vi "API_Get Current Position.vi"(10 "STATUS cluster":T1) -> (1 "Connected":bool, 3 "Probe Position":dbl)   [LabVIEW 2015, in "Tool Module.lvlib"]
doc: "Take the provided Tool Module Status cluster and extract the current axial position. Also output the current connection status. This is used to enable or disable and grayout the position display.\n\nThis vi can be used with the Tool STATUS cluster sent as the payload of the Tool Module Broadcast Event.Send Status User Event.\n\n<b>Note:</b> This VI was modified by the <b>Validate DQMH Module</b> tool to turn off automatic error handling."
uses:
  Tool Module.lvlib
  Support/_STATUS Typedef--cluster.ctl
  Tool Config/Tool Cfg.lvlib
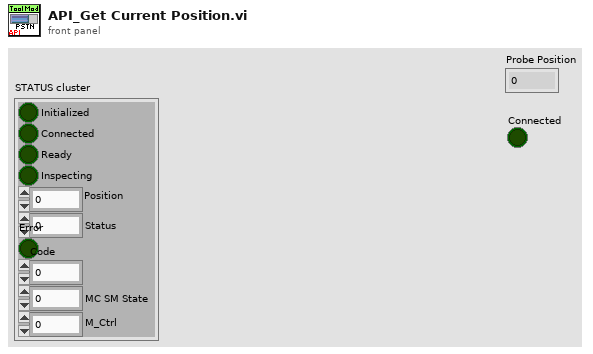
[diagram p1: front panel]
types:
  T1 = typedef "Tool Module.lvlib/_STATUS Typedef--cluster.ctl" = cluster{"Initialized":bool, "Connected":bool, "Ready":bool, "Inspecting":bool, "Position":dbl, "Status":u16, "Error":bool, "Code":i32, "MC SM State":u16, "M_Ctrl":u16}
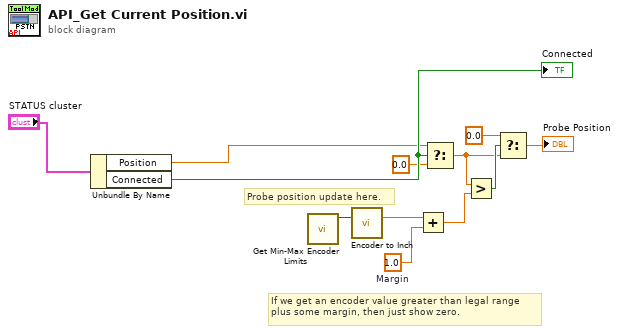
[diagram p0: block diagram]
diagram:
  w11 = 1.0  # Margin
  # "If we get an encoder value greater than legal range plus some margin, then just show zero."
  # "Probe position update here."
  n1 = Unbundle By Name("STATUS cluster") -> ("Position"=w3:dbl, "Connected"=w12:bool)
  "Connected" <- w12
  n2 = call "Get Min-Max Encoder Limits.vi"() -> ("MaxEncoder"=w2:i32)  [unwired: 8 in, 3 out]
  n3 = call "Encoder to Inch.vi"("Encoder in"=w2) -> ("Encoder out(in)"=w1:dbl)  [unwired: 14 in]
  n4 = Add(x=w1, y=w11) -> (x+y=w10:dbl)
  n5 = Select(t=w3, s=w12, f=0.0) -> (s? t:f=w6:dbl)
  n6 = Greater?(x=w6, y=w10) -> (0:w9:bool)
  n7 = Select(t=0.0, s=w9, f=w6) -> (s? t:f=→"Probe Position":dbl)
